vi "Read Analog Input with Conversion Time Module.vi"(8 "error in":errorcluster, 11 "module in":refnum<class "Module.lvclass">) -> (0 "error out":errorcluster, 1 "channel settings":T2[](array[typedef]), 2 "conversion time":T1, 3 "module out":refnum<class "Module.lvclass">)   [LabVIEW 2017, in "Scan Engine Scripting.lvlib" / "Module.lvclass"]
uses:
  Module.lvclass
  Mode Classes/Controls/analog channel settings.ctl
  Mode Classes/Analog Inputs with Conversion Time Mode/Conversion Time.ctl
  Mode Classes/Analog Inputs with Conversion Time Mode/Analog Input with Conversion Time Mode.lvclass
  C:/Users/nitest/Documents/niveristand-scan-engine-ethercat-custom-device/Custom Device Source/Scripting/Modules/Mode Classes/Analog Input Mode/Analog Input Vrms Mode/Analog Input Mode.lvclass
  Mode Classes/Analog Input Mode/Analog Input Vrms Mode/Analog Input Mode.lvclass
  Scan Engine Scripting.lvlib
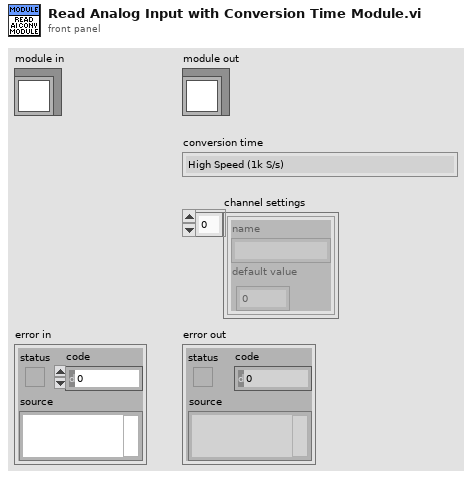
[diagram p1: front panel]
types:
  T1 = typedef "Scan Engine Scripting.lvlib/Analog Input with Conversion Time Mode.lvclass/Conversion Time.ctl" = enum16{"High Speed (1k S/s)", "Medium Speed (100 S/s)", "Medium Resolution (50/60Hz Rejection - 12 S/s)", "High Resolution (50/60Hz Rejection - 2 S/s)"}
  T2 = typedef "Scan Engine Scripting.lvlib/analog channel settings.ctl" = cluster{"name":string, "default value":dbl}
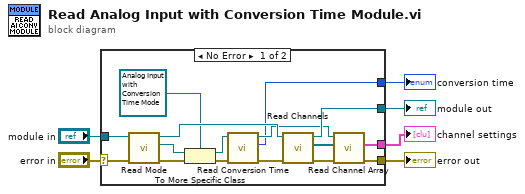
[diagram p0: block diagram]
diagram:
  n1 = case shown="No Error" "error in" {
    selector: "error in" -> [w21 w24]
    tunnel: [w14 w24] -> w3
    tunnel: [w17 w23] -> w4
    tunnel: "module in" -> [w22 w23]
    tunnel: [w12 _] -> w2
    tunnel: [w7 _] -> w1
    frame No Error {
      n2 = call-dynamic "Read Mode.vi"("error in"=w21, "module in"=w22) -> ("error out"=w19:errorcluster, "mode"=w20:refnum<class "Mode.lvclass">, "module out"=w18:refnum<class "Module.lvclass">)  [unwired: 7 in]
      n3 = To More Specific Class(target class=refnum<class "Analog Input with Conversion Time Mode.lvclass"> refnum ("Scan Engine Scripting.lvlib:Analog Input Vrms Mode.lvclass"), reference=w20, error in=w19) -> (specific class reference=w10:refnum<class "Analog Input with Conversion Time Mode.lvclass">, error out=w11:errorcluster)
      n4 = call-dynamic "Read Conversion Time.vi"("error in"=w11, "analog input with conversion time mode in"=w10) -> ("error out"=w8:errorcluster, "conversion time"=w7:T1, "analog input with conversion time mode out"=w9:refnum<class "Analog Input with Conversion Time Mode.lvclass">)  [unwired: 7 in]
      n5 = call-dynamic "Read Channels.vi"("error in"=w8, "module in"=w18) -> ("error out"=w15:errorcluster, "channels"=w13:refnum<class "Channel.lvclass">[], "module out"=w17:refnum<class "Module.lvclass">)  [unwired: 7 in]
      n6 = call "Read Channel Array.vi"("error in"=w15, "channels"=w13, "analog input mode in"=w9) -> ("error out"=w14:errorcluster, "channel settings"=w12:T2[])  [unwired: 6 in, 1 out]
    }
    frame Error {
    }
  }
  "error out" <- w3
  "module out" <- w4
  "channel settings" <- w2
  "conversion time" <- w1
